vi "Get Text Size.vi"(6 "Thickness (Default: 1)":i32=1, 7 "Text Drawing Settings (Default: Simplex)":T2={"OpenCV Font Face"=enum."FONT_HERSHEY_SIMPLEX", "Font Scale"=1.0}, 8 "error in (no error)":errorcluster, 11 "Text":string) -> (0 "error out":errorcluster, 1 "Base Line":i32, 3 "Size":T1)   [LabVIEW 2020, in "image.lvlib"]
doc: "Calculate the size the given Text will be when drawn with the specified parameters."
uses:
  image.lvlib
  Text Drawing Settings.ctl
  Font Face.ctl
  common/Image Size (Integer).ctl
  common/common.lvlib
  common/bin/gartoolkit_32-1.dll
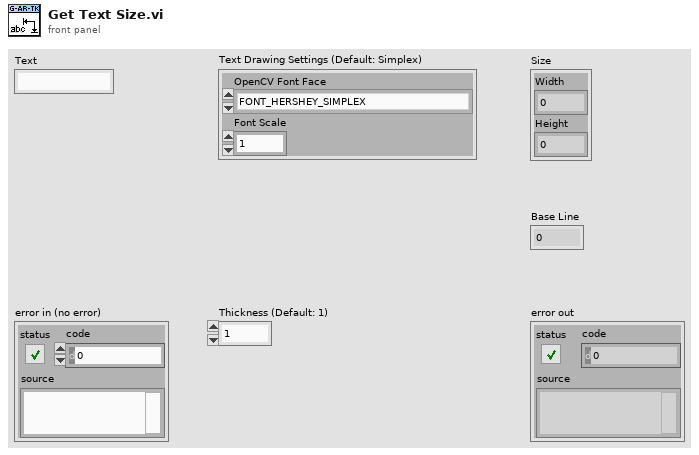
[diagram p1: front panel]
types:
  T1 = typedef "common.lvlib/Image Size (Integer).ctl" = cluster{"Width":u16, "Height":u16}
  T2 = typedef "image.lvlib/Text Drawing Settings.ctl" = cluster{"OpenCV Font Face":T3, "Font Scale":dbl}
  T3 = typedef "image.lvlib/Font Face.ctl" = enum8{"FONT_HERSHEY_SIMPLEX", "FONT_HERSHEY_PLAIN", "FONT_HERSHEY_DUPLEX", "FONT_HERSHEY_COMPLEX", "FONT_HERSHEY_TRIPLEX", "FONT_HERSHEY_COMPLEX_SMALL", "FONT_HERSHEY_SCRIPT_SIMPLEX", "FONT_HERSHEY_SCRIPT_COMPLEX", "FONT_ITALIC"}
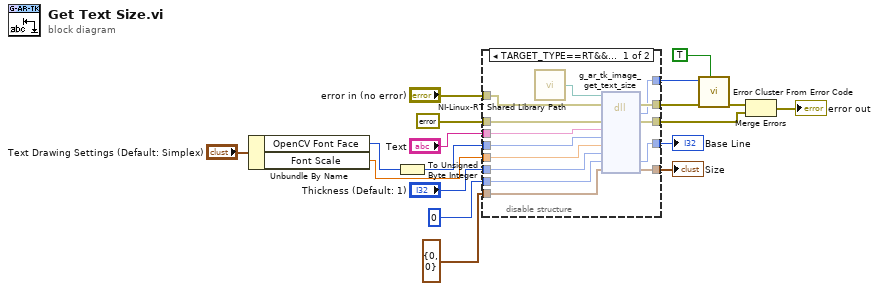
[diagram p0: block diagram]
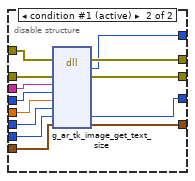
[diagram p2: hidden frame]
diagram:
  n1 = Unbundle By Name("Text Drawing Settings (Default: Simplex)") -> ("OpenCV Font Face"=w16:T3, "Font Scale"=w10:dbl)
  n2 = To Unsigned Byte Integer(number=w16) -> (unsigned 8bit integer=w11:u8)
  n3 = disable-structure shown="TARGET_TYPE==RT&&OS==Linux" {
    disable-tunnel: "error in (no error)" -> [w32 w45]
    disable-tunnel: errorcluster {"status"=FALSE, "code"=0, "source"=""} ("error constant") -> [w31 w44]
    disable-tunnel: "Text" -> [w30 w43]
    disable-tunnel: w11 -> [w29 w42]
    disable-tunnel: w10 -> [w28 w41]
    disable-tunnel: "Thickness (Default: 1)" -> [w27 w40]
    disable-tunnel: 0 ("base_line") -> [w26 w39]
    disable-tunnel: T1 {"Width"=0, "Height"=0} ("Size") -> [w25 w38]
    disable-tunnel: [w24 w37] -> w6
    disable-tunnel: [w23 w36] -> w5
    disable-tunnel: [w22 w35] -> w4
    disable-tunnel: [w21 w34] -> w3
    disable-tunnel: [w20 w33] -> w2
    frame condition #0 {
      n4 = call "NI-Linux-RT Shared Library Path.vi"() -> ("Path"=w19:path)
      n5 = dll-call lib="?" fn="g_ar_tk_image_get_text_size"(path in=w19, error in=w32, "error_cluster"=w31, "text"=w30, "font_face"=w29, "font_scale"=w28, "thickness"=w27, "base_line"=w26, "size"=w25) -> (error out=w24:errorcluster, "MgErr"=w23:i32, "error_cluster"=w22:errorcluster, "base_line"=w21:i32, "size"=w20:T1)  [unwired: 5 in, 1 out]
    }
    frame condition #1 (active) {
      n6 = dll-call lib="C:/serenial/lib/g-augmented-reality-toolkit/LabVIEW/common/bin/gartoolkit_*-1.*" fn="g_ar_tk_image_get_text_size"(error in=w45, "error_cluster"=w44, "text"=w43, "font_face"=w42, "font_scale"=w41, "thickness"=w40, "base_line"=w39, "size"=w38) -> (error out=w37:errorcluster, "MgErr"=w36:i32, "error_cluster"=w35:errorcluster, "base_line"=w34:i32, "size"=w33:T1)  [unwired: 6 in, 1 out]
    }
  }
  "Size" <- w2
  "Base Line" <- w3
  n7 = call <vilib>:"Error Cluster From Error Code.vi"("show call chain? (False)"=TRUE, "error in (no error)"=w6, "error code (0)"=w5) -> ("error out"=w15:errorcluster)  [unwired: 6 in]
  n8 = Merge Errors(w15, w4) -> (→"error out":errorcluster)
